vi "rsscope_FormatUSBPDPacketTypeInt32_ReadCallback.vi"(5 "Attribute":T1={"Identifier"="", "Descriptive Name"="", "Data Type"=enum."Integer 32", "Command"="", "Access"=enum."Read/Write", "Range Table"="", "Read Callback"="", "Write Callback"="", "Supported Models"="", "Instrument Options"="", "Index"=0, "OPC Wait"=FALSE, "No Status Check"=FALSE, "Cache Only"=FALSE}, 7 "Repeated Capability":string, 8 "error in (no error)":errorcluster, 11 "VISA resource name":refnum<visa-resource-name>) -> (0 "error out":errorcluster, 2 "Attribute Value I32":i32, 3 "VISA resource name out":refnum<visa-resource-name>)   [LabVIEW 2014]
doc: "This VI sets the attribute value.\n\nThis is a low-level VI that you can use to set the values of instrument-specific properties and inherent IVI properties. If the property represents an instrument state, this VI performs instrument I/O in the following cases:\n\n- State caching is disabled for the entire session or for the particular property.\n\n- State caching is enabled and the currently cached value is invalid or is different than the value you specify. \n\nThis instrument driver contains high-level VIs that set most of the instrument properties. It is best to use the high-level driver VIs as much as possible. They handle order dependencies and multithread locking for you. In addition, they perform status checking only after setting all of the properties. In contrast, when you set multiple properties using the SetAttribute VIs, the VIs check the instrument status after each call.\n\nAlso, when state caching is enabled, the high-level VIs that configure multiple properties perform instrument I/O only for the properties whose value you change. Thus, you can safely call the high-level VIs without the penalty of redundant instrument I/O."
uses:
  rsidr_core.llb/rsscope_rsidr_core.lvlib
  rsidr_core.llb/type_Attribute_Data_Type.ctl
  rsidr_core.llb/type_Attribute.ctl
  rsidr_core.llb/type_ReadWriteAccess.ctl
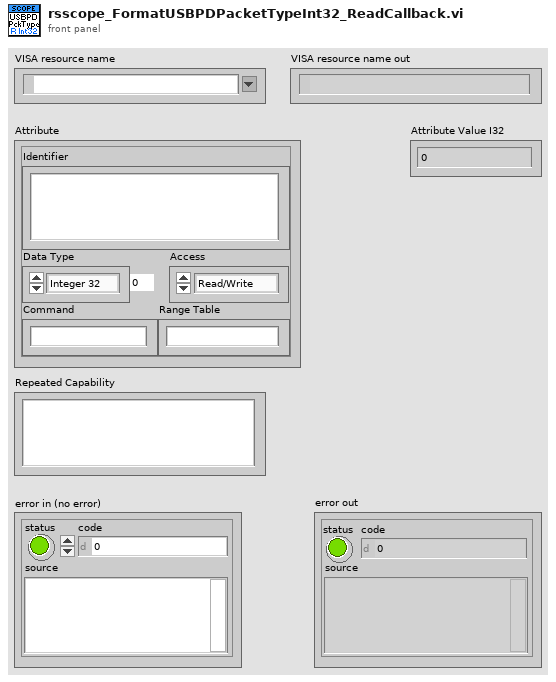
[diagram p1: front panel]
types:
  T1 = typedef "rsscope_rsidr_core.lvlib/type_Attribute.ctl" = cluster{"Identifier":string, "Descriptive Name":string, "Data Type":T2, "Command":string, "Access":T3, "Range Table":string, "Read Callback":string, "Write Callback":string, "Supported Models":string, "Instrument Options":string, "Index":i32, "OPC Wait":bool, "No Status Check":bool, "Cache Only":bool}
  T2 = typedef "rsscope_rsidr_core.lvlib/type_Attribute_Data_Type.ctl" = enum16{"Integer 32", "Double", "String", "Boolean", "None", "Integer 64", "RawString"}
  T3 = typedef "rsscope_rsidr_core.lvlib/type_ReadWriteAccess.ctl" = enum16{"Read Only", "Write Only", "Read/Write"}
  T4 = typedef "rsscope_rsidr_core.lvlib/type_Session_Data.ctl" = cluster{"IDN string":string, "Instrument FW":string, "Instr type":string, "Instr type for err. msg.":string, "Installed Options":string[], "Ignore Error Messages":string, "Logging params":variant, "OPC Timeout":i32, "VISA Timeout":i32, "STB Poll VISA Timeout":i32, "Additional Flags":i32, "Wait Before Read":i32, "Wait Before Write":i32, "Option String Flags":i32, "IO Segment Size":i64, "VISA Access Mode":T5, "Interface Type":T6, "OPC Wait Mode":T7, "Bin Float Number  Format":T8, "Bin Integer Number Format":T9, "Simulate":bool, "VXIcapable":bool, "Duplicate Session":bool, "Add LF to Write":bool, "Logging":bool, "Fast Sweep":bool, "Query Instrument Status":bool, "Check Range":bool, "Check Options":bool}
  T5 = typedef "rsscope_rsidr_core.lvlib/type_VisaAccessMode.ctl" = u16
  T6 = typedef "rsscope_rsidr_core.lvlib/type_InterfaceType.ctl" = enum16{"Unknown", "GPIB", "VXI", "GPIB_VXI", "ASRL", "PXI", "TCPIP", "USB", "SOCKET"}
  T7 = typedef "rsscope_rsidr_core.lvlib/type_OPC_Wait_Mode.ctl" = enum16{"STBpolling", "STBpollingSlow", "STBpollingSuperSlow", "ServiceRequest", "OPCquery"}
  T8 = typedef "rsscope_rsidr_core.lvlib/type_Binary_Float_Number_Format.ctl" = enum16{"Float_4_Bytes_Swapped", "Float_4_Bytes", "Double_8_Bytes_Swapped", "Double_8_Bytes"}
  T9 = typedef "rsscope_rsidr_core.lvlib/type_Binary_Integer_Number_Format.ctl" = enum16{"Int32_4_Bytes_Swapped", "Int32_4 Bytes", "Int16_2_Bytes_Swapped", "Int16_2_Bytes"}
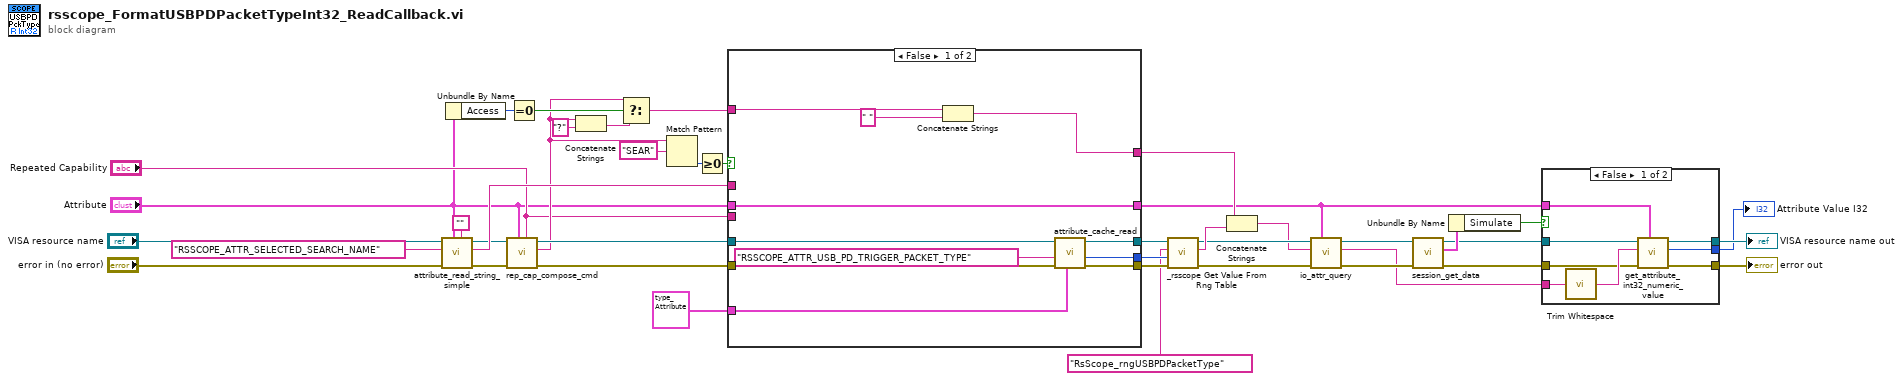
[diagram p0: block diagram]
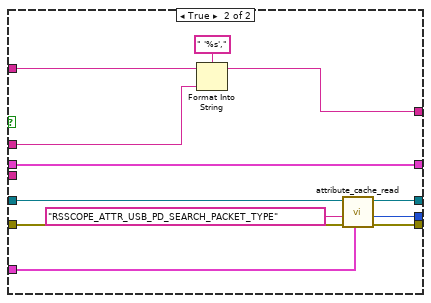
[diagram p3: hidden frame]
diagram:
  n1 = call "attribute_read_string_simple.vi"("Repeated Capability"="" ("Empty String Constant"), "Attribute"="Attribute", "error in"="error in (no error)", "Direct Attribute ID (\"\")"="RSSCOPE_ATTR_SELECTED_SEARCH_NAME" ("Direct Attribute ID (\"\")"), "VISA resource name"="VISA resource name") -> ("error out"=w39:errorcluster, "String out"=w38:string, "VISA resource name out"=w37:refnum<visa-resource-name>)  [unwired: 4 in]
  n2 = Unbundle By Name("Attribute") -> ("Access"=w33:T3)
  n3 = call "rep_cap_compose_cmd.vi"("Repeated Capability"="Repeated Capability", "Attribute"="Attribute", "error in"=w39, "VISA resource name"=w37) -> ("error out"=w29:errorcluster, "Command out"=w21:string, "VISA resource name out"=w30:refnum<visa-resource-name>)  [unwired: 5 in]
  n4 = Equal To 0?(x=w33) -> (x = 0?=w32:bool)
  n5 = Concatenate Strings(w21, "?" ("string")) -> (w35:string)
  n6 = Select(t=w21, s=w32, f=w35) -> (s? t:f=w31:string)
  n7 = Match Pattern(string=w21, regular expression="SEAR" ("true string")) -> (offset past match=w23:i32)  [unwired: 1 in, 3 out]
  n8 = Greater Or Equal To 0?(x=w23) -> (x >= 0?=w22:bool)
  n9 = case shown="False" w22 {
    tunnel: w38 -> [_ w63]
    tunnel: [w51 w62] -> w36
    tunnel: w31 -> [w52 w61]
    tunnel: w30 -> [w46 w54]
    tunnel: w29 -> [w47 w55]
    tunnel: [w44 w57] -> w28
    tunnel: [w45 w58] -> w27
    tunnel: [w43 w56] -> w26
    tunnel: "Repeated Capability" -> [_ _]
    tunnel: "Attribute" -> [w49 w60]
    tunnel: [w49 w60] -> w5
    tunnel: T1 {"Identifier"="", "Descriptive Name"="", "Data Type"=enum."Integer 32", "Command"="", "Access"=enum."Read/Write", "Range Table"="", "Read Callback"="", "Write Callback"="", "Supported Models"="", "Instrument Options"="", "Index"=0, "OPC Wait"=FALSE, "No Status Check"=FALSE, "Cache Only"=FALSE} ("Attribute") -> [w42 w53]
    frame False {
      n10 = Concatenate Strings(w52, " " ("string")) -> (w51:string)
      n11 = call "attribute_cache_read.vi"("Attribute"=w42, "error in"=w47, "Direct Attribute ID (Attribute cluster)"="RSSCOPE_ATTR_USB_PD_TRIGGER_PACKET_TYPE" ("Direct Attribute ID (\"\")"), "VISA resource name"=w46) -> ("error out"=w45:errorcluster, "Int32 out"=w43:i32, "VISA resource name out"=w44:refnum<visa-resource-name>)  [unwired: 5 out]
    }
    frame True {
      n12 = Format Into String(format string=" '%s',", initial string=w61, w63) -> (resulting string=w62:string)  [unwired: 1 in, 1 out]
      n13 = call "attribute_cache_read.vi"("Attribute"=w53, "error in"=w55, "Direct Attribute ID (Attribute cluster)"="RSSCOPE_ATTR_USB_PD_SEARCH_PACKET_TYPE" ("Direct Attribute ID (\"\")"), "VISA resource name"=w54) -> ("error out"=w58:errorcluster, "Int32 out"=w56:i32, "VISA resource name out"=w57:refnum<visa-resource-name>)  [unwired: 5 out]
    }
  }
  n14 = call "_rsscope Get Value From Rng Table.vi"("error in (no error)"=w27, "Value"=w26, "Range Table Name"="RsScope_rngUSBPDPacketType", "VISA resource name"=w28) -> ("error out"=w16:errorcluster, "Output Enum value"=w24:string, "VISA resource name out"=w15:refnum<visa-resource-name>)  [unwired: 5 in]
  n15 = Concatenate Strings(w36, w24) -> (w14:string)
  n16 = call "io_attr_query.vi"("Attribute"=w5, "error in"=w16, "write buffer"=w14, "VISA resource name"=w15) -> ("error out"=w3:errorcluster, "read buffer"=w1:string, "VISA resource name out"=w2:refnum<visa-resource-name>)  [unwired: 5 in]
  n17 = call "session_get_data.vi"("error in"=w3, "VISA resource name"=w2) -> ("error out"=w10:errorcluster, "Session User Data out"=w13:T4, "VISA resource name out"=w9:refnum<visa-resource-name>)  [unwired: 6 in, 1 out]
  n18 = Unbundle By Name(w13) -> ("Simulate"=w4:bool)
  n19 = case shown="False" w4 {
    tunnel: [w69 w74] -> w6
    tunnel: [w68 w73] -> w8
    tunnel: [w71 _] -> w7
    tunnel: w5 -> [w70 _]
    tunnel: w10 -> [w66 w74]
    tunnel: w9 -> [w65 w73]
    tunnel: w1 -> [w67 _]
    frame False {
      n20 = call <vilib>:"Trim Whitespace.vi"("string"=w67) -> ("trimmed string"=w72:string)  [unwired: 1 in]
      n21 = call "get_attribute_int32_numeric_value.vi"("Attribute"=w70, "error in"=w66, "Cmd Value in"=w72, "VISA resource name"=w65) -> ("error out"=w69:errorcluster, "Int32 value out"=w71:i32, "VISA resource name out"=w68:refnum<visa-resource-name>)  [unwired: 5 in]
    }
    frame True {
    }
  }
  "error out" <- w6
  "VISA resource name out" <- w8
  "Attribute Value I32" <- w7
